vi "Calculate Input Voltage Values.vi"(8 "error in":errorcluster, 9 "Points":i32, 10 "Voltage stop level":dbl, 11 "Voltage start level":dbl) -> (0 "error out":errorcluster, 3 "Voltage values":dbl[](array[numeric]))   [LabVIEW 2021, in "Scalar Efficiency And Load Regulation_PMIC.lvlib"]
uses:
  Scalar Efficiency And Load Regulation_PMIC.lvlib
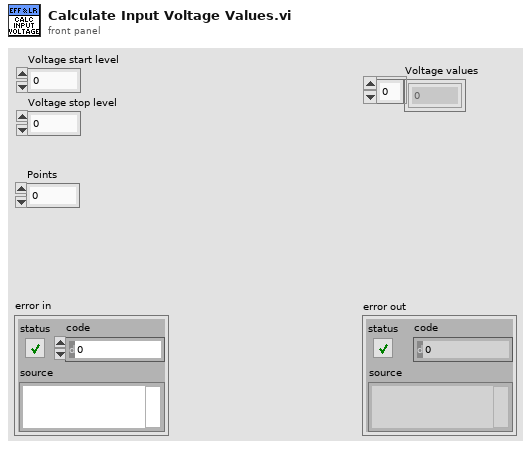
[diagram p1: front panel]
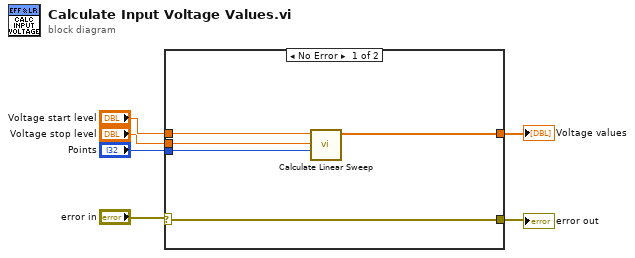
[diagram p0: block diagram]
diagram:
  n1 = case shown="No Error" "error in" {
    selector: "error in" -> [w7 w12]
    tunnel: [w11 _] -> w5
    tunnel: "Points" -> [w10 _]
    tunnel: "Voltage start level" -> [w9 _]
    tunnel: "Voltage stop level" -> [w8 _]
    tunnel: [w7 w12] -> w1
    frame No Error {
      n2 = call "Calculate Linear Sweep.vi"("Points"=w10, "Stop level"=w8, "Start level"=w9) -> ("Values"=w11:dbl[])  [unwired: 8 in]
    }
    frame Error {
    }
  }
  "Voltage values" <- w5
  "error out" <- w1
